vi "create_weights.vi"(0 "weight2":dbl[][](array[numeric]), 1 "Ring":u16(ring) items=["sensor1", "sensor 2", "sensor 3"], 2 "weight1":dbl[][](array[numeric])) -> ()   [LabVIEW 2009]
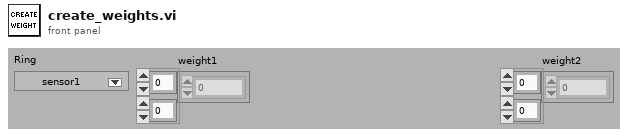
[diagram p1: front panel]
types:
  T1 = enum16{"open", "replace", "create", "open or create", "replace or create", "replace or create with confirmation"}
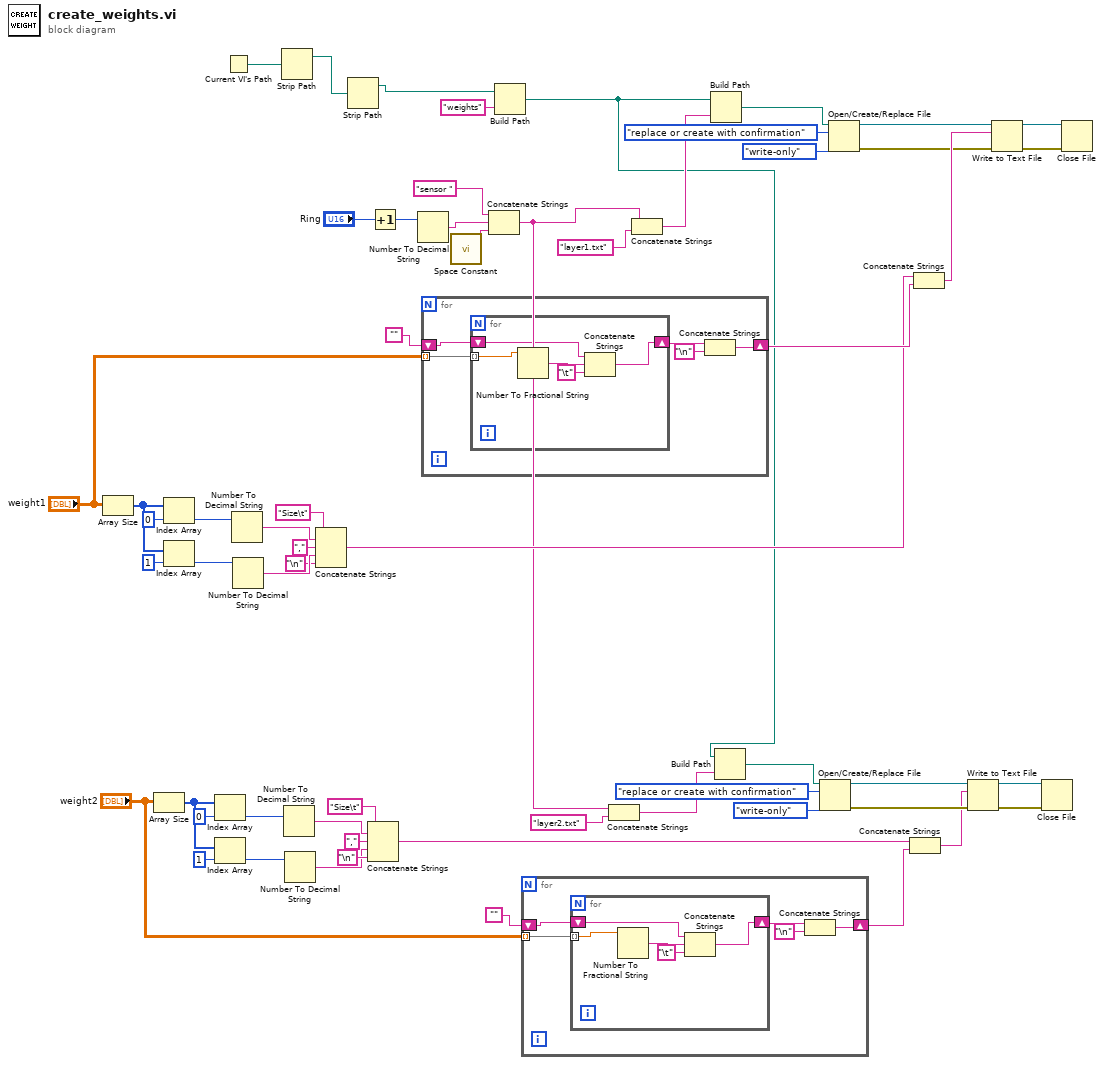
[diagram p0: block diagram]
diagram:
  n1 = Array Size(array="weight1") -> (size(s)=w43:i32[])
  n2 = Array Size(array="weight2") -> (size(s)=w24:i32[])
  n3 = Index Array(array=w43, index=0) -> (element=w41:i32)
  n4 = Index Array(array=w43, index=1) -> (element=w40:i32)
  n5 = Index Array(array=w24, index=0) -> (element=w26:i32)
  n6 = Index Array(array=w24, index=1) -> (element=w27:i32)
  n7 = Current VI's Path() -> (path=w38:path)
  n8 = Number To Decimal String(number=w41) -> (decimal integer string=w56:string)  [unwired: 1 in]
  n9 = Number To Decimal String(number=w40) -> (decimal integer string=w55:string)  [unwired: 1 in]
  n10 = Strip Path(path=w38) -> (stripped path=w2:path)  [unwired: 1 out]
  n11 = Number To Decimal String(number=w26) -> (decimal integer string=w8:string)  [unwired: 1 in]
  n12 = Number To Decimal String(number=w27) -> (decimal integer string=w9:string)  [unwired: 1 in]
  n13 = Concatenate Strings("Size\t" ("text"), w56, "," ("string"), w55, "\n" ("string")) -> (w7:string)
  n14 = Strip Path(path=w2) -> (stripped path=w1:path)  [unwired: 1 out]
  n15 = Concatenate Strings("Size\t" ("text"), w8, "," ("string"), w9, "\n" ("string")) -> (w18:string)
  n16 = Increment(x="Ring") -> (x+1=w36:u16)
  n17 = Number To Decimal String(number=w36) -> (decimal integer string=w35:string)  [unwired: 1 in]
  n18 = for {
    shift-right: [w61] -> w48
    shift-left: "" -> [w64]
    tunnel: "weight1" -> [w60] mode=indexing
    n19 = for {
      shift-right: [w66] -> w62
      shift-left: w64 -> [w67]
      tunnel: w60 -> [w65] mode=indexing
      n20 = Number To Fractional String(number=w65) -> (F-format string=w69:string)  [unwired: 3 in]
      n21 = Concatenate Strings(w67, w69, "\t" ("string")) -> (w66:string)
    }
    n22 = Concatenate Strings(w62, "\n" ("string")) -> (w61:string)
  }
  n23 = call <vilib>:"Space Constant.vi"() -> ("String"=w33:string)
  n24 = Concatenate Strings("sensor ", w35, w33) -> (w5:string)
  n25 = Build Path(base path=w1, name or relative path="weights") -> (appended path=w3:path)
  n26 = for {
    shift-right: [w71] -> w19
    shift-left: "" -> [w74]
    tunnel: "weight2" -> [w70] mode=indexing
    n27 = for {
      shift-right: [w76] -> w72
      shift-left: w74 -> [w77]
      tunnel: w70 -> [w75] mode=indexing
      n28 = Number To Fractional String(number=w75) -> (F-format string=w79:string)  [unwired: 3 in]
      n29 = Concatenate Strings(w77, w79, "\t" ("string")) -> (w76:string)
    }
    n30 = Concatenate Strings(w72, "\n" ("string")) -> (w71:string)
  }
  n31 = Concatenate Strings(w5, "layer2.txt") -> (w30:string)
  n32 = Concatenate Strings(w5, "layer1.txt") -> (w31:string)
  n33 = Build Path(base path=w3, name or relative path=w31) -> (appended path=w59:path)
  n34 = Build Path(base path=w3, name or relative path=w30) -> (appended path=w13:path)
  n35 = Open/Create/Replace File(file path (use dialog)=w13, operation (0:open)=T1."replace or create with confirmation", access (0:read/write)=enum16{"read/write", "read-only", "write-only"}."write-only") -> (refnum out=w21:refnum<file>, error out=w22:errorcluster)  [unwired: 3 in, 1 out]
  n36 = Open/Create/Replace File(file path (use dialog)=w59, operation (0:open)=T1."replace or create with confirmation", access (0:read/write)=enum16{"read/write", "read-only", "write-only"}."write-only") -> (refnum out=w46:refnum<file>, error out=w45:errorcluster)  [unwired: 3 in, 1 out]
  n37 = Concatenate Strings(w18, w19) -> (w20:string)
  n38 = Concatenate Strings(w7, w48) -> (w47:string)
  n39 = Write to Text File(file (use dialog)=w21, text=w20, error in=w22) -> (refnum out=w16:refnum<file>, error out=w17:errorcluster)  [unwired: 1 in, 1 out]
  n40 = Write to Text File(file (use dialog)=w46, text=w47, error in=w45) -> (refnum out=w50:refnum<file>, error out=w49:errorcluster)  [unwired: 1 in, 1 out]
  n41 = Close File(refnum=w16, error in=w17) -> ()  [unwired: 2 out]
  n42 = Close File(refnum=w50, error in=w49) -> ()  [unwired: 2 out]
